vi "Convert Shutdown Furnace to Heater State Enum.vi"(8 "error in (no error)":errorcluster) -> (0 "error out":errorcluster)   [LabVIEW 2018]
uses:
  Convert Shutdown Furnace to Heater State Enum-case.ctl
  Libraries/Thermal Chamber Controller_DQMH/Heater State--enum.ctl
  Libraries/Thermal Chamber Controller_DQMH/Thermal Chamber Controller_DQMH.lvlib
  <vilib>/addons/_JKI Toolkits/Caraya/classes/Assert/Assert.lvclass
  <vilib>/addons/_JKI Toolkits/Caraya/classes/Test/Test.lvclass
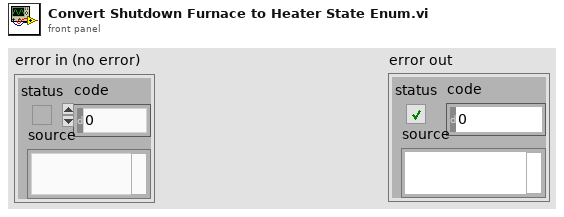
[diagram p1: front panel]
types:
  T1 = typedef "Convert Shutdown Furnace to Heater State Enum-case.ctl" = cluster{"test case ID":string, "Shutdown Furnace":bool, "Expected Heater State":T2}
  T2 = typedef "Thermal Chamber Controller_DQMH.lvlib/Heater State--enum.ctl" = enum16{"Heater Enabled", "Heater Disabled"}
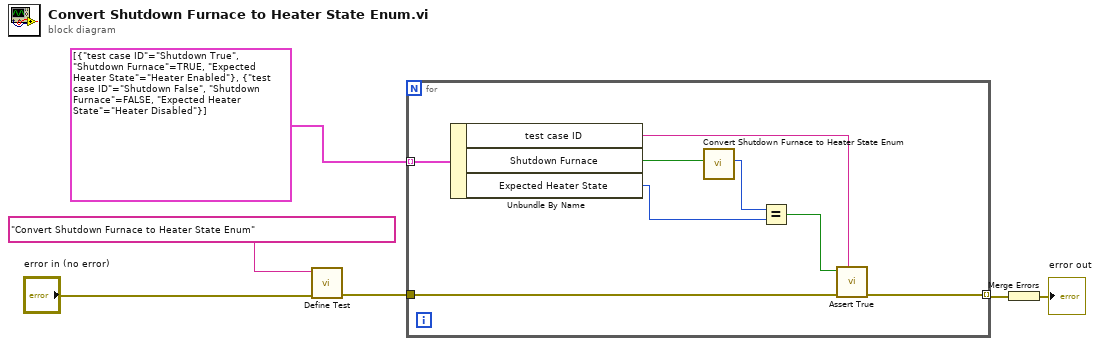
[diagram p0: block diagram]
diagram:
  n1 = call <vilib>:"Define Test.vi"("error in (no error)"="error in (no error)", "Label (VI Title)"="Convert Shutdown Furnace to Heater State Enum") -> ("error out"=w3:errorcluster)  [unwired: 9 in]
  n2 = for {
    tunnel: T1[] [{"test case ID"="Shutdown True", "Shutdown Furnace"=TRUE, "Expected Heater State"=enum."Heater Enabled"}, {"test case ID"="Shutdown False", "Shutdown Furnace"=FALSE, "Expected Heater State"=enum."Heater Disabled"}] -> [w14] mode=indexing
    tunnel: [w8] -> w5 mode=indexing
    tunnel: w3 -> [w7]
    n3 = Unbundle By Name(w14) -> ("test case ID"=w9:string, "Shutdown Furnace"=w13:bool, "Expected Heater State"=w11:T2)
    n4 = call "Convert Shutdown Furnace to Heater State Enum.vi"("Shutdown Furnace?"=w13) -> ("Heater State"=w12:T2)  [unwired: 10 in]
    n5 = Equal?(x=w12, y=w11) -> (x = y?=w10:bool)
    n6 = call <vilib>:"Assert True.vi"("Label"=w9, "error in (no error)"=w7, "True?"=w10) -> ("error out"=w8:errorcluster)  [unwired: 8 in]
  }
  n7 = Merge Errors(w5) -> (→"error out":errorcluster)
